vi "read_return_std.vi"(8 "error in (no error)":errorcluster, 11 "ARDRegression in":refnum<class "ARDRegression.lvclass">) -> (0 "error out":errorcluster, 2 "return_std":bool, 3 "ARDRegression out":refnum<class "ARDRegression.lvclass">)   [LabVIEW 2020, in "ARDRegression.lvclass"]
uses:
  ARDRegression.lvclass
  ARDRegression.lvclass/ARDRegression.ctl
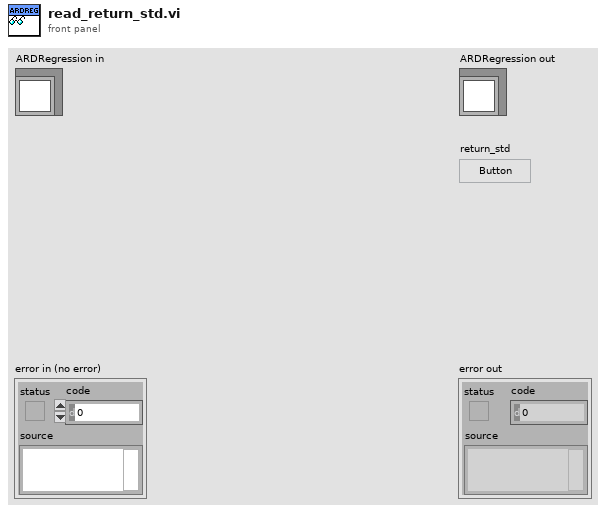
[diagram p1: front panel]
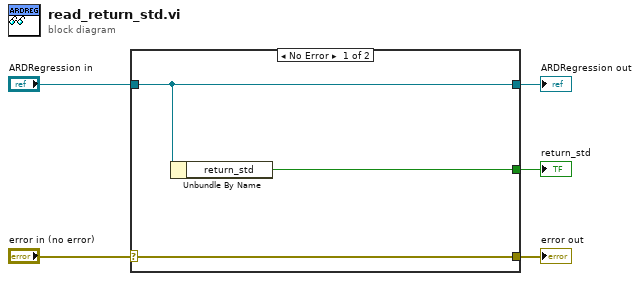
[diagram p0: block diagram]
diagram:
  n1 = case shown="No Error" "error in (no error)" {
    selector: "error in (no error)" -> [w8 w9]
    tunnel: [w8 w9] -> w4
    tunnel: [w7 w10] -> w2
    tunnel: "ARDRegression in" -> [w7 w10]
    tunnel: [w6 _] -> w1
    frame No Error {
      n2 = Unbundle By Name(w7) -> ("return_std"=w6:bool)
    }
    frame Error {
    }
  }
  "error out" <- w4
  "ARDRegression out" <- w2
  "return_std" <- w1
